vi "Dat2PosByCH.vi"(1 "RatioClusterArray":cluster{dbl, dbl}[](array[cluster]), 2 "Draw Area Size":T1) -> (0 "MappedPostionInPicture":cluster{i16, i16}[](array[cluster]))   [LabVIEW 2016]
uses:
  <vilib>/Utility/miscctls.llb/LVBoundsTypeDef.ctl
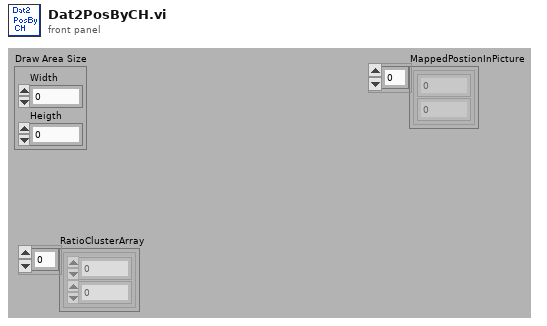
[diagram p1: front panel]
types:
  T1 = typedef "LVBoundsTypeDef.ctl" = cluster{"Width":u32, "Height":u32}
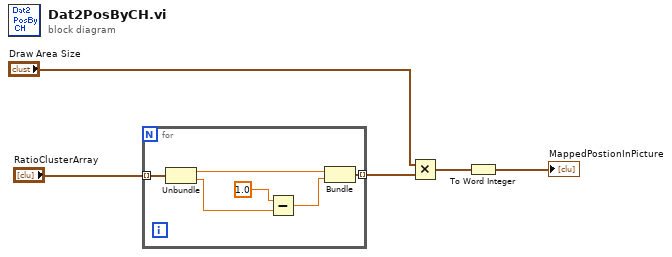
[diagram p0: block diagram]
diagram:
  n1 = for {
    tunnel: "RatioClusterArray" -> [w11] mode=indexing
    tunnel: [w7] -> w2 mode=indexing
    n2 = Unbundle(w11) -> (w10:dbl, w6:dbl)
    n3 = Subtract(x=1.0, y=w6) -> (x-y=w8:dbl)
    n4 = Bundle(w10, w8) -> (w7:cluster{dbl, dbl})  [unwired: 1 out]
  }
  n5 = Multiply(x="Draw Area Size", y=w2) -> (x*y=w1:cluster{dbl, dbl}[])
  n6 = To Word Integer(number=w1) -> (16bit integer=→"MappedPostionInPicture":cluster{i16, i16}[])
